vi "PH_IEEE1394Camera.get Basic Cam Information.vi"(0 "i ref in":refnum<vi>, 5 "error in (no error)":errorcluster) -> (14 "i ref out":refnum<vi>, 16 "IMAQ1394 Session Out":T1, 18 "Cam Error out":errorcluster, 19 "error out":errorcluster)   [LabVIEW 2014, in "PH_IEEE1394Camera.lvlib"]
doc: "This VI gets basic camara information which has to got only once and saves it to own attributes and shows it in different GUI elements."
uses:
  PH_IEEE1394Camera.lvlib
  <vilib>/userdefined/High Color/IMAQdx.ctl
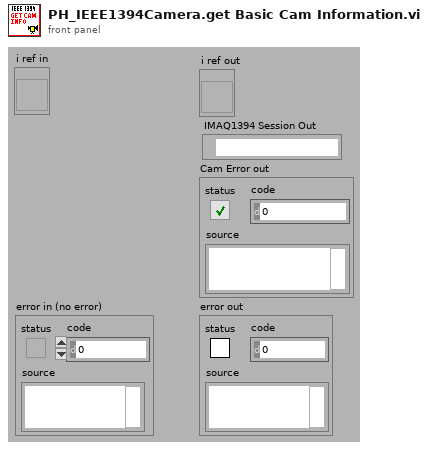
[diagram p1: front panel]
types:
  T1 = typedef "IMAQdx.ctl" = refnum<k21>
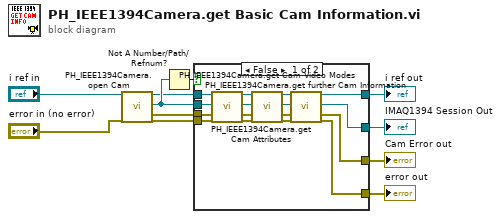
[diagram p0: block diagram]
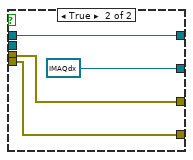
[diagram p2: hidden frame]
diagram:
  n1 = call "PH_IEEE1394Camera.open Cam.vi"("VI in"="i ref in", "error in (no error)"="error in (no error)") -> ("VI out"=w4:refnum<vi>, "Cam Session Out"=w5:T1, "Cam Error out"=w3:errorcluster, "error out"=w2:errorcluster)  [unwired: 14 in]
  n2 = Not A Number/Path/Refnum?(number/path/refnum=w5) -> (NaN/Path/Refnum?=w7:bool)
  n3 = case shown="False" w7 {
    tunnel: w4 -> [w27 w31]
    tunnel: [w15 w31] -> w9
    tunnel: [w16 w30] -> w8
    tunnel: w3 -> [w17 w29]
    tunnel: w5 -> [w20 _]
    tunnel: w2 -> [w14 w30]
    tunnel: [w13 w29] -> w6
    tunnel: [w12 T1 refnum ("IMAQ1394 Session Out")] -> w1
    frame False {
      n4 = call "PH_IEEE1394Camera.get Cam Attributes.vi"("i ref in"=w27, "IMAQ1394 Session In"=w20, "Cam Error in"=w17, "error in (no error)"=w14) -> ("i ref out"=w26:refnum<vi>, "IMAQ1394 Session Out"=w19:T1, "Cam Error out"=w18:errorcluster, "error out"=w25:errorcluster)  [unwired: 12 in]
      n5 = call "PH_IEEE1394Camera.get Cam Video Modes.vi"("i ref in"=w26, "IMAQ1394 Session In"=w19, "Cam Error in"=w18, "error in (no error)"=w25) -> ("i ref out"=w24:refnum<vi>, "IMAQ1394 Session Out"=w22:T1, "Cam Error out"=w21:errorcluster, "error out"=w23:errorcluster)  [unwired: 12 in]
      n6 = call "PH_IEEE1394Camera.get further Cam Information.vi"("i ref in"=w24, "IMAQ1394 Session In"=w22, "Cam Error in"=w21, "error in (no error)"=w23) -> ("i ref out"=w15:refnum<vi>, "IMAQ1394 Session Out"=w12:T1, "Cam Error out"=w13:errorcluster, "error out"=w16:errorcluster)  [unwired: 12 in]
    }
    frame True {
    }
  }
  "i ref out" <- w9
  "error out" <- w8
  "Cam Error out" <- w6
  "IMAQ1394 Session Out" <- w1
